vi "ARD-LTC2499_Example.vi"   [LabVIEW 2014]
doc: "This example shows how to read ADC value from LTC2499."
uses:
  PWS_ESP8266/PWS_ESP8266.lvlib
  QwaveSys_Interface/QwaveSys_Interface.lvlib
panel:
  # "Overview: Demonstrates how to read ADC data from LTC2499. This example using ARD-LTD2499 shiled that has onboard \"LTC2499\" chip, Refer at this link: http://www.iascaled.com/store/ARD-LTC2499\nRequirements: LabVIEW Full Development System,Arduino Compatible Compiler for LabVIEW,Programmable Wireless Stamp (PWS) Library.\nInstructions:\n1. Wire the ARD-LTC2499 power pins to VCC and GND and the I2C pins to the Pmod I2C interface.  Note that on an PWS board, the I2C pins are on GPIO2 (SDA) and GPIO14 (SCL) \n2. If this example has been loaded from the Arduino Compatible Compiler for LabVIEW, simply select Compile and Download.  Otherwise, open Tools>Arduino Compatible Compiler for LabVIEW in LabVIEW, then select File>Load VI, and select this VI and then Compile and Download.\n3. Open \"Serial Monitor\" by select \"Tools>Serial Monitor\" and select baud rate to 9600.\n4. Observe the data \"Temp:\" (Internal temperature of LTC2499) being print out on serial port monitor.\n5. Observe the \"CH1:\" ADC data being print out on serial port monitor.\n\n#NOTE: \nThe LTC2499 chip is a popular delta sigma 24-Bit ADC with I2C interface by Linear Technology. The chip provides either eight differential input pairs or sixteen single-ended inputs with integrated temperature sensor and oscillator. \nrefer: http://cds.linear.com/docs/en/datasheet/2499fe.pdf"
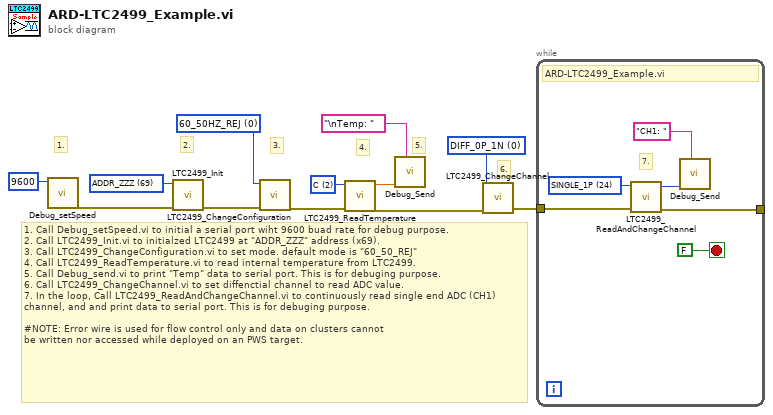
[diagram p0: block diagram]
diagram:
  w9 = u16 2 items=["K", "F", "C"] ("Temp Type")
  w3 = u16 0 items=["TEMPERATURE"=64, "SINGLE_0P"=16, "SINGLE_1P"=24, "SINGLE_2P"=17, "SINGLE_3P"=25, "SINGLE_4P"=18, "SINGLE_5P"=26, "SINGLE_6P"=19, "SINGLE_7P"=27, "SINGLE_8P"=20, "SINGLE_9P"=28, "SINGLE_10P"=21, "SINGLE_11P"=29, "SINGLE_12P"=22, "SINGLE_13P"=30, "SINGLE_14P"=23, "SINGLE_15P"=31, "DIFF_0P_1N"=0, "DIFF_2P_3N"=1, "DIFF_4P_5N"=2, "DIFF_6P_7N"=3, "DIFF_8P_9N"=4, "DIFF_10P_11N"=5, "DIFF_12P_13N"=6, "DIFF_14P_15N"=7, "DIFF_1P_0N"=8, "DIFF_3P_2N"=9, "DIFF_5P_4N"=10, "DIFF_7P_6N"=11, "DIFF_9P_8N"=12, "DIFF_11P_10N"=13, "DIFF_13P_12N"=14, "DIFF_15P_14N"=15] ("Channel")
  w10 = u16 0 items=["60_50HZ_REJ"=0, "60HZ_REJ"=32, "50HZ_REJ"=16, "SPEED_2X"=8] ("Config")
  w12 = u8 69 items=["ADDR_000"=20, "ADDR_00Z"=21, "ADDR_001"=22, "ADDR_0Z0"=23, "ADDR_0ZZ"=36, "ADDR_0Z1"=37, "ADDR_010"=38, "ADDR_01Z"=39, "ADDR_011"=40, "ADDR_Z00"=53, "ADDR_Z01"=55, "ADDR_Z0Z"=54, "ADDR_ZZ0"=68, "ADDR_ZZZ"=69, "ADDR_ZZ1"=70, "ADDR_Z10"=71, "ADDR_Z1Z"=84, "ADDR_Z11"=85, "ADDR_100"=86, "ADDR_10Z"=87, "ADDR_101"=100, "ADDR_1Z0"=101, "ADDR_1ZZ"=102, "ADDR_1Z1"=103, "ADDR_110"=116, "ADDR_111"=117, "ADDR_11Z"=118] ("Address")
  # "6."
  # "5."
  # "4."
  # "3."
  # "2."
  # "1."
  # "1. Call Debug_setSpeed.vi to initial a serial port wiht 9600 buad rate for debug purpose.\n2. Call LTC2499_Init.vi to initialzed LTC2499 at \"ADDR_ZZZ\" address (x69).\n3. Call LTC2499_ChangeConfiguration.vi to set mode. default mode is \"60_50_REJ\"\n4. Call LTC2499_ReadTemperature.vi to read internal temperature from LTC2499.\n5. Call Debug_send.vi to print \"Temp\" data to serial port. This is for debuging purpose.\n6. Call LTC2499_ChangeChannel.vi to set diffenctial channel to read ADC value.\n7. In the loop, Call LTC2499_ReadAndChangeChannel.vi to continuously read single end ADC (CH1) channel, and and print data to serial port. This is for debuging purpose.\n\n#NOTE: Error wire is used for flow control only and data on clusters cannot\nbe written nor accessed while deployed on an PWS target."
  n1 = call "Debug_setSpeed.vi"("Speed"=u32 9600) -> ("error out"=w5:errorcluster)  [unwired: 10 in]
  n2 = call "LTC2499_Init.vi"("error in (no error)"=w5, "Address"=w12) -> ("error out"=w11:errorcluster)  [unwired: 9 in]
  n3 = call "LTC2499_ChangeConfiguration.vi"("error in (no error)"=w11, "Config"=w10) -> ("error out"=w4:errorcluster)  [unwired: 9 in]
  n4 = call "LTC2499_ReadTemperature.vi"("error in (no error)"=w4, "Temp Type"=w9) -> ("error out"=w1:errorcluster, "Data"=w8:dbl)  [unwired: 8 in]
  n5 = call "Debug_Send.vi"("Name"="\nTemp: ", "DATA"=w8) -> ()  [unwired: 10 in]
  n6 = call "LTC2499_ChangeChannel.vi"("error in (no error)"=w1, "Channel"=w3) -> ("error out"=w2:errorcluster)  [unwired: 9 in]
  n7 = while {
    tunnel: w2 -> [w16]
    tunnel: [w13] -> _
    stop <- FALSE stop-if-true
    w14 = u16 24 items=["TEMPERATURE"=64, "SINGLE_0P"=16, "SINGLE_1P"=24, "SINGLE_2P"=17, "SINGLE_3P"=25, "SINGLE_4P"=18, "SINGLE_5P"=26, "SINGLE_6P"=19, "SINGLE_7P"=27, "SINGLE_8P"=20, "SINGLE_9P"=28, "SINGLE_10P"=21, "SINGLE_11P"=29, "SINGLE_12P"=22, "SINGLE_13P"=30, "SINGLE_14P"=23, "SINGLE_15P"=31, "DIFF_0P_1N"=0, "DIFF_2P_3N"=1, "DIFF_4P_5N"=2, "DIFF_6P_7N"=3, "DIFF_8P_9N"=4, "DIFF_10P_11N"=5, "DIFF_12P_13N"=6, "DIFF_14P_15N"=7, "DIFF_1P_0N"=8, "DIFF_3P_2N"=9, "DIFF_5P_4N"=10, "DIFF_7P_6N"=11, "DIFF_9P_8N"=12, "DIFF_11P_10N"=13, "DIFF_13P_12N"=14, "DIFF_15P_14N"=15] ("Next Channel")
    # "7."
    # "ARD-LTC2499_Example.vi"
    n8 = call "LTC2499_ReadAndChangeChannel.vi"("error in (no error)"=w16, "Next Channel"=w14) -> ("error out"=w13:errorcluster, "Data"=w15:i32)  [unwired: 8 in]
    n9 = call "Debug_Send.vi"("Name"="CH1: ", "DATA"=w15) -> ()  [unwired: 10 in]
  }
